vi "rsaGo.vi"(2 "error in":errorcluster, 4 "Trace length":i32) -> (0 "error out":errorcluster, 1 "traceData out":sgl[](graph)=[-35.222816, -81.97218, -75.48918, -83.79996, -83.29207, -82.89071, -81.88148, -83.53415, -82.70661, -72.54573, -82.9634, -82.29361, -81.31203, -83.01113, -82.56769, -82.87589, -83.67036, -83.36195, -72.33946, -82.59927, -84.73103, -83.97651, -83.411514, -85.18569, -82.039345, -67.94831, -83.01549, -81.9395, -83.92526, -81.17082, -81.49894, -79.75899, -78.99845, -79.988556, -81.14951, -77.37991, -81.78985, -79.529686, -80.78456, -80.805275, -80.07417, -79.3274, -80.26451, -78.6932, -81.05735, -73.9402, -83.809784, -81.09811, -78.47523, -80.26894, -80.594826, -65.73996, -80.452354, -79.41825, -80.65693, -82.849976, -75.11627, -80.48689, -79.398895, -82.59754, -76.84035, -81.77888, -62.83766, -80.05829, -80.908745, -79.16077, -81.43459, -78.868576, -85.32578, -83.00017, -81.26839, -80.762566, -82.085106, -80.59251, -82.31843, -81.98923, -81.05028, -82.16544, -66.14161, -81.77522, -81.47244, -81.219574, -81.17923, -81.55601, -81.91089, -80.12973, -81.42529, -82.00245, -80.85411, -74.67726, -82.69054, -82.480965, -80.97957, -80.33004, -81.38634, -79.55955, -81.51721, -81.54454, -84.38653, -80.44304, -81.477066, -81.41962, -83.312256, -80.82275, -76.26092, -52.669685, -82.97263, -81.11401, -83.193146, -83.092255, -83.91312, -77.361755, -81.45047, -83.79237, -81.86669, -74.733826, -82.55489, -83.90423, -80.40291, -81.94447, -84.08119, -81.43277, -80.80228, -83.05707, -83.01213, -82.02101, -82.168304, -81.66236, -85.54734, -82.353096, -80.745514, -71.136055, -82.39969, -83.60506, -79.48099, -77.83868, -80.158875, -83.108505, -68.12434, -82.29863, -80.75247, -80.46822, -74.70592, -79.873314, -78.64372, -80.64462, -84.091385, -80.20089, -81.26395, -79.858284, -82.30362, -81.64331, -81.044914, -79.1398, -80.79141, -78.44673, -81.81007, -80.80376, -59.573326, -80.80545, -80.89944, -81.7015, -82.690506, -82.02678, -75.021675, -55.26719, -81.75185, -82.66061, -80.48062, -80.003265, -79.67121, -82.15674, -81.41443, -81.43394, -81.10786, -78.13148, -82.41014, -81.95156, -78.17542, -81.52226, -81.83903, -82.71748, -82.92291, -80.79201, -79.852264, -64.158745, -79.865074, -81.696396, -80.76888, -81.75557, -81.79272, -44.194927, -67.53936, -79.68408, -81.89579, -79.99539, -83.77777, -82.69055, -82.0522, -83.364044, -82.25388, -81.08509, -80.60031, -79.41629, -79.09552, -81.77772, -82.636406, -83.00375, -80.494, -81.31687, -81.44619, -67.28499, -78.951126, -81.80029, -79.57225, -78.477715, -74.51615, -67.369675, -35.078453, -67.779175, -76.30497, -78.614876, -80.41022, -80.63707, -80.58238, -77.2235, -82.3851, -79.34964, -80.565475, -71.669205, -79.654724, -82.06148, -81.94585, -80.436264, -80.65904, -80.402435, -75.93858, -80.51324, -79.03192, -78.71421, -77.2419, -75.87307, -74.42772, -67.67462, -50.477867, -28.629349, -65.402275, -72.5892, -75.67036, -78.96194, -79.18567, -73.01126, -79.101906, -79.504616, -78.9148, -79.591736, -80.391624, -78.30125, -78.58302, -78.860596, -82.77858, -80.8289, -81.11574, -80.0093, -82.48989, -76.394455, -79.271515, -81.44924, -80.45776, -74.57824, -71.83857, -35.309982, -63.084465, -75.830925, -78.01634, -80.136536, -79.399704, -78.45105, -78.899605, -81.861404, -81.102104, -78.97264, -76.84761, -79.69739, -81.99401, -74.155, -79.40323, -78.7782, -80.98485, -77.206985, -79.95895, -70.52151, -80.50656, -77.58899, -78.338196, -73.87348, -74.006256, -58.93689, -29.066978, -60.99221, -73.27491, -74.02675, -77.7982, -77.17042, -79.46827, -70.53753, -78.78655, -79.78455, -81.95746, -79.62678, -83.07164, -76.05732, -80.263916, -82.44412, -80.58544, -81.4556, -80.76648, -81.61656, -77.65233, -79.053055, -78.99725, -78.72531, -76.821175, -73.92787, -56.02735, -34.426918, -73.96385, -77.00622, -78.16536, -80.45561, -78.414246, -68.3249, -80.55513, -79.73433, -80.53054, -80.92563, -80.92937, -78.18213, -81.76758, -79.07152, -82.51568, -80.21507, -81.72142, -82.441864, -81.842865, -80.04213, -79.05448, -79.821655, -82.30102, -80.53137, -79.00345, -44.17888, -65.18417, -80.42757, -81.67198, -77.853134, -79.57385, -78.05836, -64.01773, -80.04162, -79.04655, -80.77055, -80.25874, -79.1851, -79.35013, -80.27614, -81.041, -81.17295, -83.59801, -81.87874, -81.83669, -80.48618, -80.5909, -80.761604, -81.42142, -79.741425, -82.558685, -81.24566, -56.101166, -80.08394, -82.31131, -79.62129, -79.49703, -80.58946, -80.11835, -61.24861, -79.10618, -80.00014, -79.41455, -79.880035, -80.714645, -79.221954, -83.71576, -81.40077, -82.47858, -72.82273, -82.26065, -82.66458, -81.723206, -81.094894, -79.82444, -80.29587, -82.97322, -80.39368, -82.25009, -70.14927, -80.477356, -82.32526, -79.62251, -82.23135, -82.098175, -71.74454, -80.74486, -81.77036, -81.14192, -82.59811, -84.98046, -81.800446, -81.64158, -80.9368, -82.76462, -83.85375, -82.03209, -80.77487, -81.94191, -82.49168, -80.51352, -84.77868, -79.89177, -80.45874, -81.61011, -83.00942, -77.74364, -83.574646, -82.54157, -80.429504, -83.1926, -82.67655, -56.997917, -81.06208, -81.276505, -80.89026, -82.997055, -83.505615, -81.74982, -81.63342, -80.90942, -82.64992, -81.92758, -81.39488, -80.82877, -82.034035, -80.217476, -80.530945, -81.09564, -79.130325, -79.712616, -79.802505, -81.383095, -80.85129, -81.04289, -79.37216, -79.8699, -80.933, -77.920006, -70.58532, -81.2741, -82.24707, -80.65973, -81.418304, -81.32933, -81.31466, -81.19638, -82.297356, -78.63284, -80.55367, -84.332344, -81.373764, -81.56401, -79.41036, -81.777275, -81.266846, -81.75673, -81.80988, -84.25453, -82.70608, -80.71805, -82.16661, -82.848885, -81.23654, -81.51053, -70.07887, -82.49338, -82.15923, -80.51444, -80.9978, -81.2225, -82.84305, -80.8978, -81.731705, -81.87817, -81.635826, -80.50185, -80.35201, -83.1517, -82.00507, -78.438, -80.76828, -78.70917, -81.92674, -81.33796, -82.46541, -82.022125, -82.0805, -81.28966, -83.01093, -82.97121, -83.28767, -77.34394, -81.69496, -84.272606, -80.239, -82.101685, -82.213295, -81.87801, -77.073296, -82.769104, -79.83673, -81.344055, -83.55091, -80.89076, -80.999725, -82.67463, -79.693665, -83.34874, -82.364494, -81.48713, -82.714455, -83.20652, -81.72307, -80.70206, -82.553925, -82.762726, -77.49991, -80.84484, -79.20027, -81.838524, -81.2334, -82.397644, -81.26794, -83.56181, -78.55282, -81.06143, -82.92192, -83.15949, -84.06287, -83.21646, -82.7895, -82.37639, -82.07674, -79.73517, -80.93327, -76.97379, -78.53769, -78.97452, -79.58892, -78.5366, -80.38272, -79.85452, -79.67943, -81.41559, -80.96367, -81.2114, -82.26658, -81.15075, -80.93988, -81.25595, -81.54876, -82.75304, -81.33437, -81.22654, -80.63812, -80.55802, -80.14718, -78.20714, -81.618416, -80.805275, -82.92327, -81.53809, -81.49212, -79.30586, -80.53565, -81.64551, -83.264275, -79.723015, -80.680954, -79.06897, -81.63514, -81.06833, -78.81623, -78.84343, -80.87737, -80.90514, -80.73134, -79.22099, -72.27342, -79.274796, -81.76391, -81.72061, -80.47885, -82.04461, -83.71128, -80.74626, -79.05045, -82.20999, -81.41199, -80.20333, -80.96393, -81.84368, -81.791595, -82.2792, -81.487686, -83.01851, -78.95651, -84.21292, -81.06286, -81.49459, -81.32451, -82.37602, -83.12263, -81.982834, -83.22036, -82.29315, -81.03171, -82.62577, -81.84655, -81.262436, -82.9292, -82.02246, -83.5199, -82.530556, -82.14367, -80.611, -79.8864, -81.68964, -82.9798, -82.06745, -79.13046, -81.80603, -82.99423, -81.833664, -82.24819, -82.06962, -79.00569, -82.5437, -81.68701, -80.97676, -80.44397, -82.40798, -83.74071, -81.57301, -80.21529, -80.36971, -80.62703, -83.13393, -82.28856, -81.28605, -81.02485, -79.22533, -79.014984, -80.28655, -79.550514, -81.613846, -82.21292, -80.795944, -81.19815, -80.677376, -81.31424, -81.84918, -80.08244, -79.21073, -80.567635, -81.32827, -84.03484, -83.373276, -80.39285, -81.93859, -80.17975, -80.97896, -82.02904, -80.12369, -81.49761, -80.86546, -81.86905, -78.88908, -81.65697, -81.643135, -82.30301, -81.34805, -82.521484, -81.85871, -83.18053, -81.46992, -83.025215, -80.67255, -82.78032, -81.27707, -81.45598, -81.734886, -80.8144, -81.70467, -81.47335, -82.46408, -80.559494, -81.10968, -81.09129, -80.35817, -82.16197, -81.93164, -83.67952, -80.96824, -81.34448, -81.456604, -80.75698, -80.64848, -82.17433, -80.92934, -82.0192, -81.66551, -85.14439, -80.25656, -84.517944, -81.20426, -80.88479, -82.805466, -84.90562, -80.435074, -82.17844, -79.231865, -81.56986, -82.485275, -82.611176, -82.512665, -82.62869, -79.84821, -81.36113, -80.22142, -80.31478, -82.04566, -81.379166, -83.721886, -80.81549, -81.300285, -80.42334, -81.58311, -80.49057, -83.027916, -81.86439, -81.63632, -81.93137, -81.93091, -80.94331, -79.74123, -82.80252, -81.24788, -81.341324, -82.58966, -79.33737, -82.09901, -81.54555, -80.078415, -83.037094, -83.36659, -82.37911, -78.74238, -82.155594, -80.39421, -81.0841, -83.73555, -82.26876, -81.91616, -82.745804, -82.427704, -81.69696, -83.4476, -81.47205, -82.08881, -81.26921, -80.6532, -82.876366, -82.987335, -81.59508, -84.46062, -81.04595, -80.94014, -82.63202, -80.44514, -83.16545, -80.534805, -82.40486, -91.03313])   [LabVIEW 2016]
uses:
  <userlib>/RSA_API/RSA_API.lvlib
panel:
  in  "Trace number":u32(ring) items=["SpectrumTrace1", "SpectrumTrace2", "SpectrumTrace3"]
  out "Trace Ready":bool=TRUE
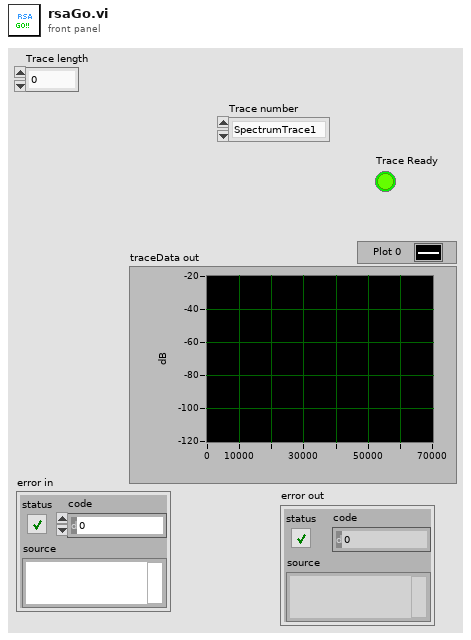
[diagram p1: front panel]
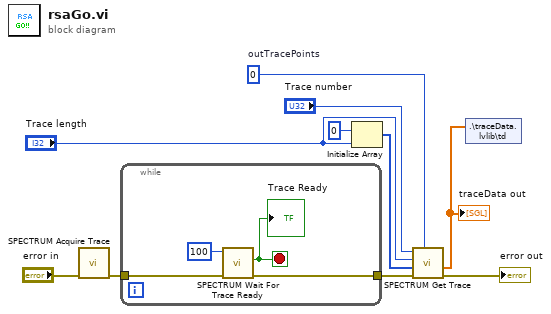
[diagram p0: block diagram]
diagram:
  w5 = 0  # outTracePoints
  n1 = call <userlib>:"SPECTRUM Acquire Trace.vi"("error in (no error)"="error in") -> ("error out"=w7:errorcluster)  [unwired: 9 in, 1 out]
  n2 = while {
    tunnel: w7 -> [w12]
    tunnel: [w11] -> w1
    stop <- w13 stop-if-true
    n3 = call <userlib>:"SPECTRUM Wait For Trace Ready.vi"("error in (no error)"=w12, "timeoutMsec"=100) -> ("error out"=w11:errorcluster, "ready out"=w13:bool)  [unwired: 7 in, 1 out]
    "Trace Ready" <- w13
  }
  n4 = Initialize Array(0 ("element"), "Trace length") -> (w3:i32[])
  n5 = call "SPECTRUM Get Trace.vi"("outTracePoints"=w5, "error in (no error)"=w1, "traceData"=w3, "maxTracePoints"="Trace length", "trace"="Trace number") -> ("error out"=→"error out":errorcluster, "traceData out"=w2:sgl[])  [unwired: 3 in, 2 out]
  "traceData out" <- w2
  n6 = shared-variable ".\\traceData.lvlib\\td"(w2) -> ()  [unwired: 1 in, 1 out]
